vi "XYZ.vi"(0 "AXIS":u16(ring) items=["X", "Y", "Z"], 1 "XYZ COM":refnum<visa-resource-name>="COM12", 5 "Set speed (r/min)":dbl=50.0, 9 "Set location (mm)":dbl=100.0, 11 "emergency stop":bool) -> (4 "X running":bool, 6 "Y running":bool, 8 "Z running":bool, 10 "Read location (mm)":dbl, 14 "error out":errorcluster)   [LabVIEW 2023]
uses:
  <vilib>/NI/Modbus Library/API/Wrapper/Create Serial Master.vi
  <vilib>/NI/Modbus Library/API/master/Modbus Master.lvclass
  <vilib>/NI/Modbus Library/API/Wrapper/API Main.lvlib
panel:
  out "coils":bool[](array[boolean])
  in  "unit ID":u8
  # "需要十六进制换算成十进制\n十进制脉冲数10000等于一圈\n如显示4E20表示十进制的20000脉冲数，对应电机转两圈\n30D40对应200000，电机转20圈"
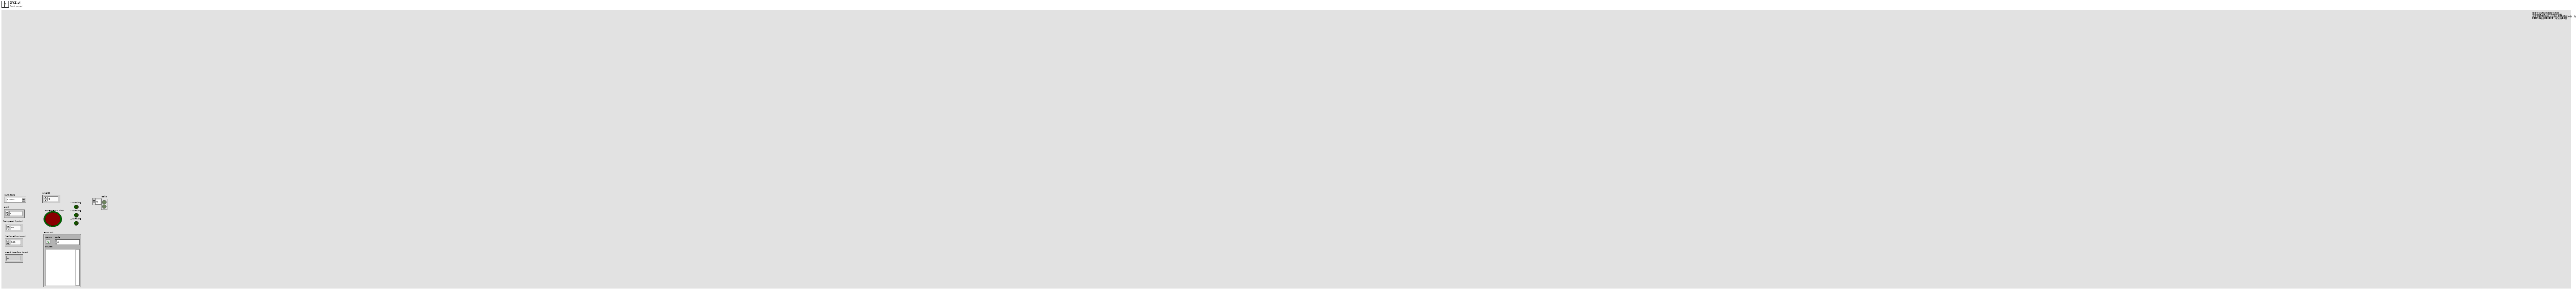
[diagram p1: front panel]
types:
  T1 = cluster{"register values[0]":u16, "register values[1]":u16}
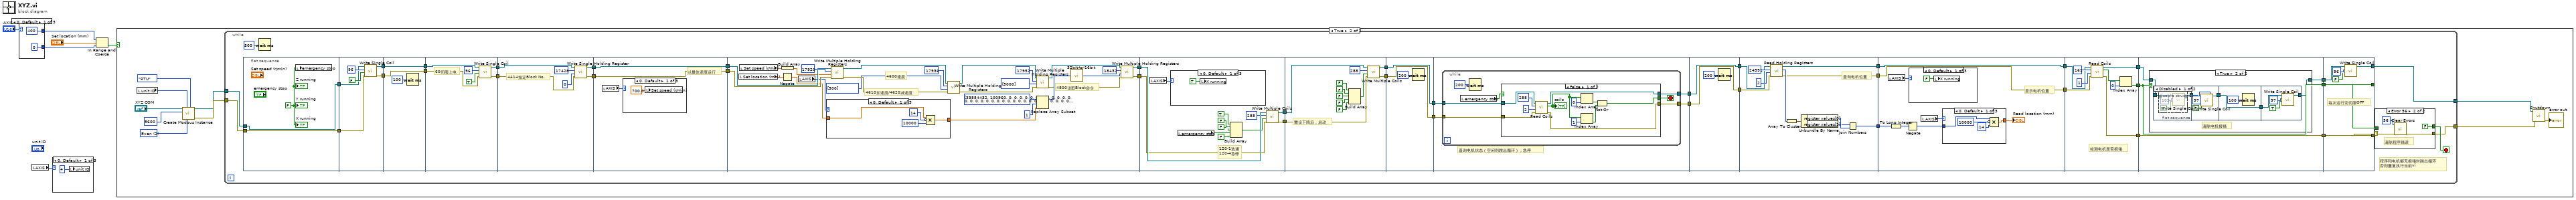
[diagram p0: block diagram]
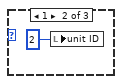
[diagram p2: hidden frame]
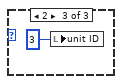
[diagram p3: hidden frame]
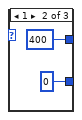
[diagram p4: hidden frame]
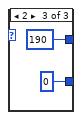
[diagram p5: hidden frame]
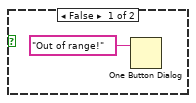
[diagram p6: hidden frame]
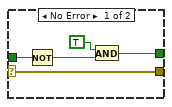
[diagram p7: hidden frame]
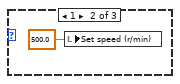
[diagram p8: hidden frame]
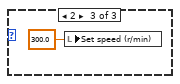
[diagram p9: hidden frame]
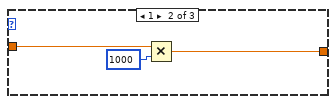
[diagram p10: hidden frame]
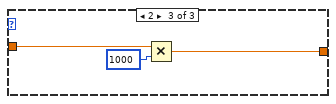
[diagram p11: hidden frame]
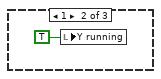
[diagram p12: hidden frame]
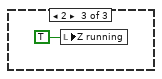
[diagram p13: hidden frame]
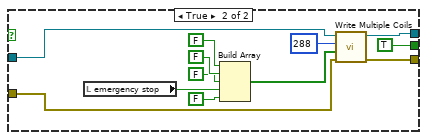
[diagram p14: hidden frame]
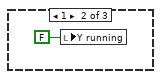
[diagram p15: hidden frame]
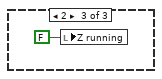
[diagram p16: hidden frame]
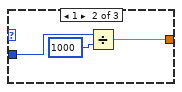
[diagram p17: hidden frame]
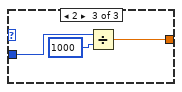
[diagram p18: hidden frame]
diagram:
  n1 = case shown="0, Default" "AXIS" {
    tunnel: [400 ("upper limit") 400 ("upper limit") 190 ("upper limit")] -> w5
    tunnel: [0 ("lower limit") 0 ("lower limit") 0 ("lower limit")] -> w4
    frame 0, Default {
    }
    frame 1 {
    }
    frame 2 {
    }
  }
  n2 = local read "AXIS"() -> (w1:u16)
  n3 = case shown="0, Default" w1 {
    frame 0, Default {
      n4 = local write "unit ID"(u8 4 ("unit ID")) -> ()
    }
    frame 1 {
      n5 = local write "unit ID"(u8 2 ("unit ID")) -> ()
    }
    frame 2 {
      n6 = local write "unit ID"(u8 3 ("unit ID")) -> ()
    }
  }
  n7 = In Range and Coerce(upper limit=w5, x="Set location (mm)", lower limit=w4) -> (In Range?=w2:bool)  [unwired: 1 out]
  n8 = case shown="True" w2 {
    frame False {
      n9 = One Button Dialog(message="Out of range!") -> ()  [unwired: 1 in, 1 out]
    }
    frame True {
      w23 = u16 2 items=["None", "Odd", "Even", "Mark", "Space"] ("parity (even)")
      n10 = local read "unit ID"() -> (w26:u8)
      n11 = call-poly <vilib>:"Create Modbus Instance.vi"("serial type"=enum16{"RTU", "ASCII"}."RTU", "parity (even)"=w23, "unit ID"=w26, "baud rate"=u32 9600, "VISA resource name"="XYZ COM") -> ("error out"=w21:errorcluster, "serial master instance"=w20:refnum<class "Modbus Master.lvclass">)  [unwired: 5 in]
      n12 = while {
        tunnel: w21 -> [w36]
        tunnel: w20 -> [w37]
        tunnel: [w40] -> w19
        tunnel: [w39] -> w18
        stop <- w51 stop-if-true
        # "程序和电机都无报错时跳出循环\n否则重复执行当前vi"
        n13 = flat-sequence {
          tunnel: w37 -> [w80]
          tunnel: w36 -> [w79]
          tunnel: [w80] -> w35
          tunnel: [w79] -> w34
          tunnel: [w85] -> w33
          tunnel: [w84] -> w31
          tunnel: w35 -> [w83]
          tunnel: w34 -> [w82]
          tunnel: w33 -> [w90]
          tunnel: [w90] -> w32
          tunnel: w31 -> [w89]
          tunnel: [w89] -> w30
          tunnel: [w94] -> w68
          tunnel: [w95] -> w69
          tunnel: w32 -> [w96]
          tunnel: w30 -> [w91]
          tunnel: [w102] -> w67
          tunnel: [w101] -> w66
          tunnel: w69 -> [w98]
          tunnel: w68 -> [w99]
          tunnel: w67 -> [w105]
          tunnel: [w105] -> w65
          tunnel: w66 -> [w104]
          tunnel: [w104] -> w64
          tunnel: w65 -> [w124]
          tunnel: w64 -> [w125]
          tunnel: [w120] -> w63
          tunnel: [w121] -> w62
          tunnel: w63 -> [w156]
          tunnel: [w154] -> w49
          tunnel: w62 -> [w155]
          tunnel: [w145] -> w48
          tunnel: w49 -> [w170]
          tunnel: [w162] -> w61
          tunnel: [w161] -> w60
          tunnel: w48 -> [w160]
          tunnel: w61 -> [w173]
          tunnel: [w173] -> w59
          tunnel: w60 -> [w172]
          tunnel: [w172] -> w58
          tunnel: w59 -> [w177]
          tunnel: [w175] -> w57
          tunnel: w58 -> [w176]
          tunnel: [w174] -> w56
          tunnel: w57 -> [w211]
          tunnel: [w211] -> w55
          tunnel: w56 -> [w210]
          tunnel: [w210] -> w54
          tunnel: [w216] -> w53
          tunnel: w55 -> [w214]
          tunnel: w54 -> [w215]
          tunnel: [w213] -> w52
          tunnel: [w212] -> w45
          tunnel: w53 -> [w224]
          tunnel: w52 -> [w229]
          tunnel: [w224] -> w47
          tunnel: [w223] -> w46
          tunnel: w45 -> [w223]
          tunnel: w47 -> [w250]
          tunnel: w46 -> [w249]
          tunnel: [w246] -> w43
          tunnel: [w245] -> w42
          tunnel: [w244] -> w41
          tunnel: w43 -> [w255]
          tunnel: w42 -> [w253]
          tunnel: w41 -> [w256]
          tunnel: [w256] -> w29
          tunnel: [w254] -> w28
          tunnel: [w253] -> w27
          tunnel: [w283] -> w38
          tunnel: [w279] -> w40
          tunnel: [w284] -> w44
          tunnel: w29 -> [w284]
          tunnel: w28 -> [w280]
          tunnel: w27 -> [w283]
          frame #0 {
            w81 = FALSE ("Y running")
            n14 = local write "emergency stop"(w81) -> ()
            "X running" <- w81
            "Y running" <- w81
            "Z running" <- w81
          }
          frame #1 {
            n15 = call-dynamic "Write Single Coil.vi"("error in"=w82, "coil to write"=FALSE, "address"=u16 96, "Modbus master in"=w83) -> ("error out"=w84:errorcluster, "Modbus master out"=w85:refnum<class "Modbus Master.lvclass">)  [unwired: 6 in]
          }
          frame #2 {
            n16 = Wait (ms)(milliseconds to wait=u32 100) -> ()  [unwired: 1 out]
          }
          frame #3 {
            # "60伺服上电"
            n17 = call-dynamic "Write Single Coil.vi"("error in"=w91, "coil to write"=TRUE, "address"=u16 96, "Modbus master in"=w96) -> ("error out"=w95:errorcluster, "Modbus master out"=w94:refnum<class "Modbus Master.lvclass">)  [unwired: 6 in]
          }
          frame #4 {
            # "4414指定Block No."
            n18 = call-dynamic "Write Single Holding Register.vi"("error in"=w98, "register to write"=u16 0, "address"=u16 17428, "Modbus master in"=w99) -> ("error out"=w101:errorcluster, "Modbus master out"=w102:refnum<class "Modbus Master.lvclass">)  [unwired: 6 in]
          }
          frame #5 {
            # "以最佳速度运行"
            n19 = local read "AXIS"() -> (w103:u16)
            n20 = case shown="0, Default" w103 {
              frame 0, Default {
                n21 = local write "Set speed (r/min)"(700.0 ("Set speed (r/min)")) -> ()
              }
              frame 1 {
                n22 = local write "Set speed (r/min)"(500.0 ("Set speed (r/min)")) -> ()
              }
              frame 2 {
                n23 = local write "Set speed (r/min)"(300.0 ("Set speed (r/min)")) -> ()
              }
            }
          }
          frame #6 {
            # "4600速度"
            # "4610加速度/4620减速度"
            # "4800读取Block命令"
            n24 = local read "Set location (mm)"() -> (w110:dbl)
            n25 = local read "Set speed (r/min)"() -> (w114:dbl)
            n26 = Negate(x=w110) -> (-x=w109:dbl)
            n27 = Build Array(w114) -> (w113:dbl[])
            n28 = local read "AXIS"() -> (w111:u16)
            n29 = case shown="0, Default" w111 {
              tunnel: w109 -> [w138 w141 w143]
              tunnel: [w135 w139 w142] -> w112
              frame 0, Default {
                n30 = Compound Arithmetic op=MULTIPLY(w138, invert 14 ("new element/subarray"), 10000 ("new element/subarray")) -> (w135:dbl)
              }
              frame 1 {
                n31 = Multiply(x=w141, y=1000) -> (x*y=w139:dbl)
              }
              frame 2 {
                n32 = Multiply(x=w143, y=1000) -> (x*y=w142:dbl)
              }
            }
            n33 = call-dynamic "Write Multiple Holding Registers.vi"("error in"=w125, "registers to write"=w113, "starting address"=u16 17920, "Modbus master in"=w124) -> ("error out"=w134:errorcluster, "Modbus master out"=w132:refnum<class "Modbus Master.lvclass">)  [unwired: 6 in]
            n34 = call-dynamic "Write Multiple Holding Registers.vi"("error in"=w134, "registers to write"=u16[] [500] ("Block动作加速度（0-20000）"), "starting address"=u16 17936, "Modbus master in"=w132) -> ("error out"=w133:errorcluster, "Modbus master out"=w131:refnum<class "Modbus Master.lvclass">)  [unwired: 6 in]
            n35 = call-dynamic "Write Multiple Holding Registers.vi"("error in"=w133, "registers to write"=u16[] [5000] ("Block动作减速度（0-20000）"), "starting address"=u16 17952, "Modbus master in"=w131) -> ("error out"=w115:errorcluster, "Modbus master out"=w116:refnum<class "Modbus Master.lvclass">)  [unwired: 6 in]
            n36 = Replace Array Subset(array=i32[] [33554432, 100960, 0, 0, 0, 0, 0, 0, 0, 0, 0, 0, 0, 0, 0, 0, 0, 0, 0, 0, 0, 0, 0, 0, 0, 0, 0, 0, 0, 0, 0, 0, 0, 0, 0, 0, 0, 0, 0, 0, 0, 0, 0, 0, 0, 0, 0, 0, 0, 0] ("y轴block输入"), new element=w112, index=1) -> (w117:i32[])
            n37 = call "32bit-to-16bit.vi"("32位寄存器值"=w117) -> ("16位寄存器值"=w123:u16[])
            n38 = call-dynamic "Write Multiple Holding Registers.vi"("error in"=w115, "registers to write"=w123, "starting address"=u16 18432, "Modbus master in"=w116) -> ("error out"=w121:errorcluster, "Modbus master out"=w120:refnum<class "Modbus Master.lvclass">)  [unwired: 6 in]
          }
          frame #7 {
            # "120-1选通\n120-4急停"
            n39 = local read "AXIS"() -> (w146:u16)
            n40 = case shown="0, Default" w146 {
              frame 0, Default {
                n41 = local write "X running"(TRUE ("Y running")) -> ()
              }
              frame 1 {
                n42 = local write "Y running"(TRUE ("Y running")) -> ()
              }
              frame 2 {
                n43 = local write "Z running"(TRUE ("Y running")) -> ()
              }
            }
            n44 = local read "emergency stop"() -> (w147:bool)
            n45 = Build Array(TRUE ("120h"), FALSE, FALSE ("122h"), w147, FALSE ("124h")) -> (w150:bool[])
            n46 = call-dynamic "Write Multiple Coils.vi"("error in"=w155, "coils to write"=w150, "starting address"=u16 288, "Modbus master in"=w156) -> ("error out"=w145:errorcluster, "Modbus master out"=w154:refnum<class "Modbus Master.lvclass">)  [unwired: 6 in]
          }
          frame #8 {
            # "需设下降沿，启动"
            n47 = Build Array(FALSE ("120h"), FALSE, FALSE ("122h 2"), FALSE ("123h 2"), FALSE ("124h 2")) -> (w165:bool[])
            n48 = call-dynamic "Write Multiple Coils.vi"("error in"=w160, "coils to write"=w165, "starting address"=u16 288, "Modbus master in"=w170) -> ("error out"=w161:errorcluster, "Modbus master out"=w162:refnum<class "Modbus Master.lvclass">)  [unwired: 6 in]
          }
          frame #9 {
            n49 = Wait (ms)(milliseconds to wait=u32 200) -> ()  [unwired: 1 out]
          }
          frame #10 {
            # "查询电机状态（空闲则跳出循环）；急停"
            n50 = while {
              tunnel: w177 -> [w183]
              tunnel: w176 -> [w182]
              tunnel: [w181] -> w175
              tunnel: [w180] -> w174
              stop <- w179 stop-if-true
              n51 = local read "emergency stop"() -> (w178:bool)
              n52 = Wait (ms)(milliseconds to wait=u32 200) -> ()  [unwired: 1 out]
              n53 = case shown="False" w178 {
                tunnel: w183 -> [w193 w201]
                tunnel: w182 -> [w192 w200]
                tunnel: [w191 w199] -> w181
                tunnel: [w190 w198] -> w180
                tunnel: [w185 TRUE] -> w179
                frame False {
                  n54 = call-dynamic "Read Coils.vi"("error in"=w192, "number of inputs"=u16 2, "starting address"=u16 258, "Modbus master in"=w193) -> ("error out"=w190:errorcluster, "coils"=w188:bool[], "Modbus master out"=w191:refnum<class "Modbus Master.lvclass">)  [unwired: 5 in]
                  "coils" <- w188
                  n55 = Index Array(array=w188, index=0) -> (element=w187:bool)
                  n56 = Index Array(array=w188, index=1) -> (element=w186:bool)
                  n57 = Not Or(1:w186, 2:w187) -> (0:w185:bool)
                }
                frame True {
                  n58 = local read "emergency stop"() -> (w208:bool)
                  n59 = Build Array(FALSE ("120h"), FALSE, FALSE ("122h"), w208, FALSE ("124h")) -> (w207:bool[])
                  n60 = call-dynamic "Write Multiple Coils.vi"("error in"=w200, "coils to write"=w207, "starting address"=288, "Modbus master in"=w201) -> ("error out"=w198:errorcluster, "Modbus master out"=w199:refnum<class "Modbus Master.lvclass">)  [unwired: 6 in]
                }
              }
            }
          }
          frame #11 {
            n61 = Wait (ms)(milliseconds to wait=u32 200) -> ()  [unwired: 1 out]
          }
          frame #12 {
            # "查询电机位置"
            n62 = call-dynamic "Read Holding Registers.vi"("error in"=w215, "number of inputs"=u16 2 ("number of holding registers"), "starting address"=u16 24591, "Modbus master in"=w214) -> ("error out"=w216:errorcluster, "register values"=w222:u16[], "Modbus master out"=w212:refnum<class "Modbus Master.lvclass">)  [unwired: 5 in]
            n63 = Array To Cluster(array=w222) -> (cluster=w219:T1)
            n64 = Unbundle By Name(w219) -> ("register values[0]"=w218:u16, "register values[1]"=w217:u16)
            n65 = Join Numbers(hi=w217, lo=w218) -> ((hi.lo)=w213:u32)
          }
          frame #13 {
            # "显示电机位置"
            n66 = local read "AXIS"() -> (w227:u16)
            n67 = To Long Integer(number=w229) -> (32bit integer=w226:i32)
            n68 = Negate(x=w226) -> (-x=w225:i32)
            n69 = case shown="0, Default" w227 {
              frame 0, Default {
                n70 = local write "X running"(FALSE ("Y running")) -> ()
              }
              frame 1 {
                n71 = local write "Y running"(FALSE ("Y running")) -> ()
              }
              frame 2 {
                n72 = local write "Z running"(FALSE ("Y running")) -> ()
              }
            }
            n73 = local read "AXIS"() -> (w228:u16)
            n74 = case shown="0, Default" w228 {
              tunnel: [w235 w238 w241] -> w230
              tunnel: w225 -> [w234 w240 w242]
              frame 0, Default {
                n75 = Compound Arithmetic op=MULTIPLY(w234, invert 10000, 14) -> (w235:dbl)
              }
              frame 1 {
                n76 = Divide(x=w240, y=1000) -> (x/y=w238:dbl)
              }
              frame 2 {
                n77 = Divide(x=w242, y=1000) -> (x/y=w241:dbl)
              }
            }
            "Read location (mm)" <- w230
          }
          frame #14 {
            # "检测电机是否报错"
            n78 = call-dynamic "Read Coils.vi"("error in"=w250, "number of inputs"=u16 1, "starting address"=u16 161, "Modbus master in"=w249) -> ("error out"=w244:errorcluster, "coils"=w247:bool[], "Modbus master out"=w246:refnum<class "Modbus Master.lvclass">)  [unwired: 5 in]
            n79 = Index Array(array=w247, index=0) -> (element=w245:bool)
          }
          frame #15 {
            n80 = case shown="True" w253 {
              tunnel: w255 -> [w257 w260]
              tunnel: [w257 w262] -> w254
              frame False {
              }
              frame True {
                # "清除电机报错"
                n81 = flat-sequence {
                  tunnel: [w264] -> w259
                  tunnel: w260 -> [w263]
                  tunnel: w259 -> [w270]
                  tunnel: [w269] -> w258
                  tunnel: w258 -> [w274]
                  tunnel: [w274] -> w261
                  tunnel: w261 -> [w276]
                  tunnel: [w275] -> w262
                  frame #0 {
                    n82 = disable-structure shown="Disabled" {
                      disable-tunnel: [w266 _] -> w264
                      disable-tunnel: w263 -> [w265 _]
                      frame Disabled {
                        n83 = call-dynamic "Write Single Coil.vi"("coil to write"=FALSE, "address"=u16 103 ("starting address"), "Modbus master in"=w265) -> ("Modbus master out"=w266:refnum<class "Modbus Master.lvclass">)  [unwired: 7 in, 1 out]
                      }
                      frame Enabled {
                      }
                    }
                  }
                  frame #1 {
                    n84 = call-dynamic "Write Single Coil.vi"("coil to write"=FALSE, "address"=u16 97 ("starting address"), "Modbus master in"=w270) -> ("Modbus master out"=w269:refnum<class "Modbus Master.lvclass">)  [unwired: 7 in, 1 out]
                  }
                  frame #2 {
                    n85 = Wait (ms)(milliseconds to wait=u32 100) -> ()  [unwired: 1 out]
                  }
                  frame #3 {
                    n86 = call-dynamic "Write Single Coil.vi"("coil to write"=TRUE, "address"=u16 97 ("starting address"), "Modbus master in"=w276) -> ("Modbus master out"=w275:refnum<class "Modbus Master.lvclass">)  [unwired: 7 in, 1 out]
                  }
                }
              }
            }
          }
          frame #16 {
            # "每次运行完伺服OFF"
            n87 = call-dynamic "Write Single Coil.vi"("coil to write"=FALSE, "address"=u16 96 ("starting address"), "Modbus master in"=w280) -> ("Modbus master out"=w279:refnum<class "Modbus Master.lvclass">)  [unwired: 7 in, 1 out]
          }
        }
        n88 = Wait (ms)(milliseconds to wait=u32 500) -> ()  [unwired: 1 out]
        n89 = case shown="Error 56" w44 {
          selector: w44 -> [w74 w77]
          tunnel: [w70 FALSE] -> w51
          tunnel: [w74 w75] -> w39
          tunnel: w38 -> [w73 _]
          frame No Error {
            n90 = Not(x=w73) -> (.not. x?=w72:bool)
            n91 = And(x=TRUE, y=w72) -> (x .and. y?=w70:bool)
          }
          frame Error {
            # "清除程序错误"
            n92 = call <vilib>:"Clear Errors.vi"("error in (no error)"=w77, "specific error code to clear (0: all)"=56) -> ("error out"=w75:errorcluster)  [unwired: 4 in, 1 out]
          }
        }
      }
      n93 = call-dynamic "Shutdown.vi"("error in"=w18, "Modbus master in"=w19) -> ("error out"=→"error out":errorcluster)  [unwired: 9 in]
    }
  }
